vi "实时小时数据处理整合 (子VI).vi"(11 "枚举":enum16{"实时数据排序", "小时数据排序"}(ring)) -> (3 "已排序的数组":string[](array[string]))   [LabVIEW 2016, in "数据传输系统.lvlib"]
uses:
  <userlib>/_OpenG.lib/array/array.llb/Remove Duplicates from 1D Array (String)__ogtk.vi
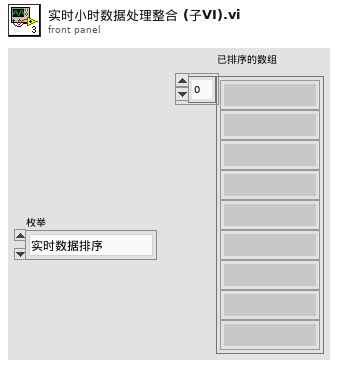
[diagram p1: front panel]
types:
  T1 = cluster{"PH":string[][], "CODCr":string[][], "氨氮":string[][], "CODMn":string[][], "总氮":string[][], "总磷":string[][], "电导率":string[][], "水温":string[][], "COD":string[][], "DO":string[][], "浊度":string[][], "叶绿素":string[][], "藻密度":string[][], "铜":string[][], "盐度":string[][], "水位":string[][], "流速":string[][], "方向":string[][], "瞬时流量":string[][], "累积流量":string[][], "正累积流量":string[][], "负累积流量":string[][], "亚硝酸盐":string[][], "硫化物":string[][], "ORP":string[][], "铅":string[][], "镉":string[][], "锌":string[][], "镍":string[][], "锰":string[][], "汞":string[][], "气温":string[][], "气压":string[][], "风速":string[][], "风向":string[][], "空气温度":string[][], "相对湿度":string[][], "分钟雨量":string[][], "小时雨量":string[][], "日雨量":string[][], "累积雨量":string[][], "盐度":string[][], "磷酸盐":string[][], "硝氮":string[][], "氟化物":string[][], "挥发酚":string[][], "氯化物":string[][], "蓝绿藻":string[][], "余氯":string[][], "综合生物毒性":string[][], "水深":string[][]}
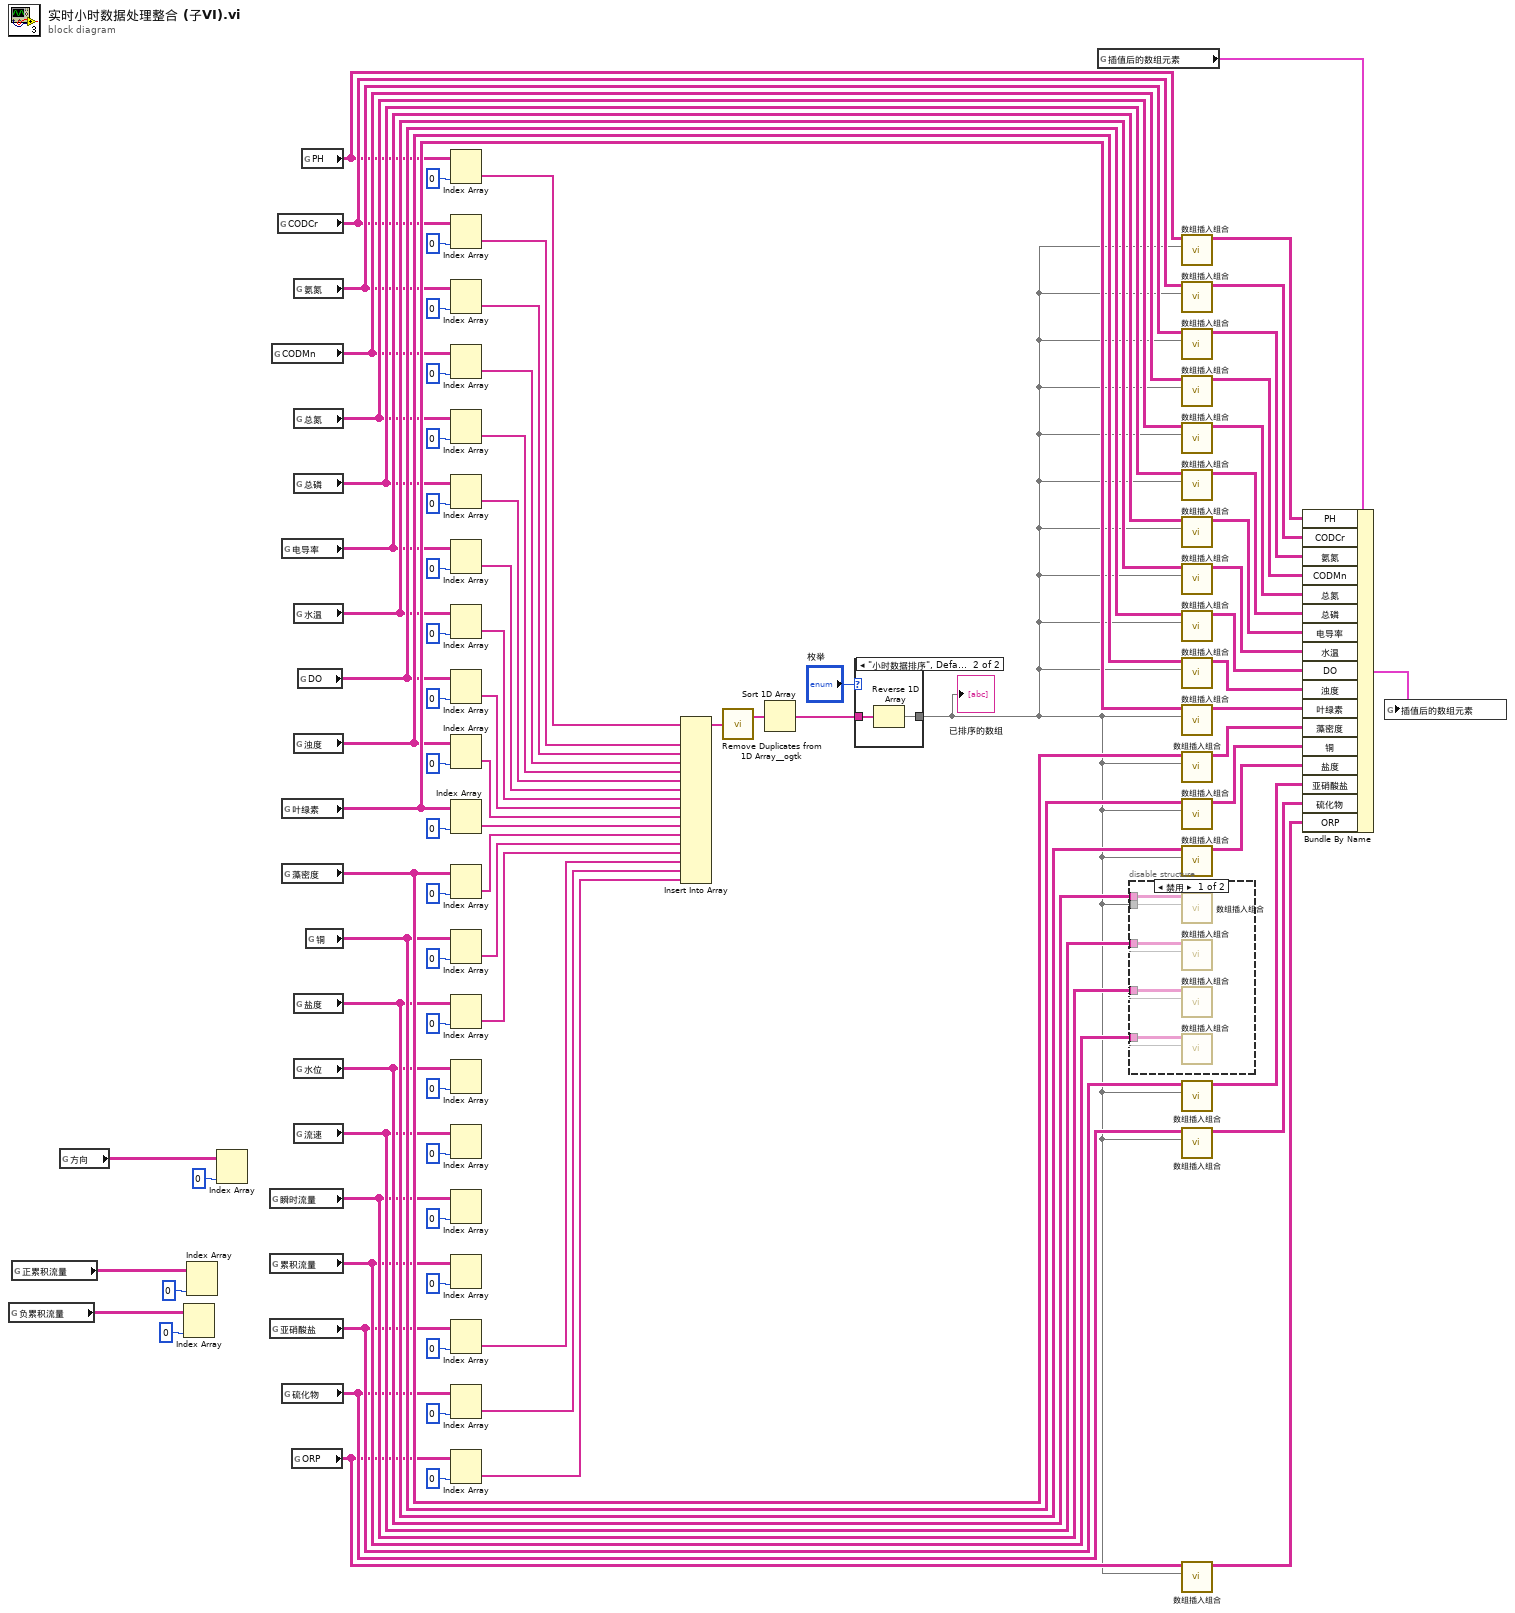
[diagram p0: block diagram]
diagram:
  n1 = global read "全局 所有参数.vi" "负累积流量"() -> (w5:string[][])
  n2 = global read "全局 所有参数.vi" "正累积流量"() -> (w6:string[][])
  n3 = global read "全局 所有参数.vi" "方向"() -> (w9:string[][])
  n4 = Index Array(array=w5, index (col)=0 ("索引 (列)")) -> ()  [unwired: 1 in, 1 out]
  n5 = Index Array(array=w6, index (col)=0 ("索引 (列)")) -> ()  [unwired: 1 in, 1 out]
  n6 = Index Array(array=w9, index (col)=0 ("索引 (列)")) -> ()  [unwired: 1 in, 1 out]
  n7 = global read "全局 所有参数.vi" "瞬时流量"() -> (w23:string[][])
  n8 = global read "全局 所有参数.vi" "累积流量"() -> (w22:string[][])
  n9 = global read "全局 所有参数.vi" "亚硝酸盐"() -> (w19:string[][])
  n10 = global read "全局 所有参数.vi" "CODMn"() -> (w70:string[][])
  n11 = global read "全局 所有参数.vi" "CODCr"() -> (w68:string[][])
  n12 = global read "全局 所有参数.vi" "电导率"() -> (w73:string[][])
  n13 = global read "全局 所有参数.vi" "叶绿素"() -> (w77:string[][])
  n14 = global read "全局 所有参数.vi" "藻密度"() -> (w78:string[][])
  n15 = global read "全局 所有参数.vi" "硫化物"() -> (w16:string[][])
  n16 = global read "全局 所有参数.vi" "ORP"() -> (w15:string[][])
  n17 = global read "全局 所有参数.vi" "氨氮"() -> (w69:string[][])
  n18 = global read "全局 所有参数.vi" "总氮"() -> (w71:string[][])
  n19 = global read "全局 所有参数.vi" "总磷"() -> (w72:string[][])
  n20 = global read "全局 所有参数.vi" "水温"() -> (w74:string[][])
  n21 = global read "全局 所有参数.vi" "浊度"() -> (w76:string[][])
  n22 = global read "全局 所有参数.vi" "盐度"() -> (w36:string[][])
  n23 = global read "全局 所有参数.vi" "水位"() -> (w28:string[][])
  n24 = global read "全局 所有参数.vi" "流速"() -> (w26:string[][])
  n25 = global read "全局 所有参数.vi" "DO"() -> (w75:string[][])
  n26 = global read "全局 所有参数.vi" "PH"() -> (w66:string[][])
  n27 = global read "全局 所有参数.vi" "铜"() -> (w37:string[][])
  n28 = Index Array(array=w66, index (col)=0 ("索引 (行)")) -> (element=w53:string[])  [unwired: 1 in]
  n29 = Index Array(array=w68, index (col)=0 ("索引 (行)")) -> (element=w54:string[])  [unwired: 1 in]
  n30 = Index Array(array=w69, index (col)=0 ("索引 (行)")) -> (element=w55:string[])  [unwired: 1 in]
  n31 = Index Array(array=w70, index (col)=0 ("索引 (行)")) -> (element=w56:string[])  [unwired: 1 in]
  n32 = Index Array(array=w71, index (col)=0 ("索引 (行)")) -> (element=w57:string[])  [unwired: 1 in]
  n33 = Index Array(array=w72, index (col)=0 ("索引 (行)")) -> (element=w58:string[])  [unwired: 1 in]
  n34 = Index Array(array=w73, index (col)=0 ("索引 (行)")) -> (element=w59:string[])  [unwired: 1 in]
  n35 = Index Array(array=w74, index (col)=0 ("索引 (行)")) -> (element=w60:string[])  [unwired: 1 in]
  n36 = Index Array(array=w75, index (col)=0 ("索引 (行)")) -> (element=w61:string[])  [unwired: 1 in]
  n37 = Index Array(array=w76, index (col)=0 ("索引 (行)")) -> (element=w62:string[])  [unwired: 1 in]
  n38 = Index Array(array=w77, index (col)=0 ("索引 (行)")) -> (element=w63:string[])  [unwired: 1 in]
  n39 = Index Array(array=w78, index (col)=0 ("索引 (行)")) -> (element=w64:string[])  [unwired: 1 in]
  n40 = Index Array(array=w37, index (col)=0 ("索引 (行)")) -> (element=w35:string[])  [unwired: 1 in]
  n41 = Index Array(array=w36, index (col)=0 ("索引 (行)")) -> (element=w34:string[])  [unwired: 1 in]
  n42 = Index Array(array=w28, index (col)=0 ("索引 (列)")) -> ()  [unwired: 1 in, 1 out]
  n43 = Index Array(array=w26, index (col)=0 ("索引 (列)")) -> ()  [unwired: 1 in, 1 out]
  n44 = Index Array(array=w23, index (col)=0 ("索引 (列)")) -> ()  [unwired: 1 in, 1 out]
  n45 = Index Array(array=w22, index (col)=0 ("索引 (列)")) -> ()  [unwired: 1 in, 1 out]
  n46 = Index Array(array=w19, index (col)=0 ("索引 (列)")) -> (element=w3:string[])  [unwired: 1 in]
  n47 = Index Array(array=w16, index (col)=0 ("索引 (列)")) -> (element=w2:string[])  [unwired: 1 in]
  n48 = Index Array(array=w15, index (col)=0 ("索引 (列)")) -> (element=w1:string[])  [unwired: 1 in]
  n49 = Insert Into Array(array=w53, new element #1=w54, new element #2=w55, new element #3=w56, new element #4=w57, new element #5=w58, new element #6=w59, new element #7=w60, new element #8=w61, new element #9=w62, new element #10=w63, new element #11=w64, new element #12=w35, new element #13=w34, new element #14=w3, new element #15=w2, new element #16=w1) -> (w65:string[])  [unwired: 1 in]
  n50 = call-poly <userlib>:"Remove Duplicates from 1D Array__ogtk.vi"("Input Array"=w65) -> ("Output Array"=w52:string[])  [unwired: 1 out]
  n51 = Sort 1D Array(array=w52) -> (sorted array=w38:string[])
  n52 = case shown="\"小时数据排序\", Default" "枚举" {
    tunnel: w38 -> [w90 w92]
    tunnel: [w90 w91] -> w12
    frame "实时数据排序" {
    }
    frame "小时数据排序", Default {
      n53 = Reverse 1D Array(array=w92) -> (reversed array=w91:string[])
    }
  }
  "已排序的数组" <- w12
  n54 = global read "插值后的新数组.vi" "插值后的数组元素"() -> (w21:T1)
  n55 = disable-structure shown="禁用" {
    disable-tunnel: w28 -> [w97 _]
    disable-tunnel: w26 -> [w96 _]
    disable-tunnel: w23 -> [w95 _]
    disable-tunnel: w22 -> [w94 _]
    disable-tunnel: w12 -> [w93 _]
    frame Disabled {
      n56 = call "数组插入组合.vi"("排序后的一维数组"=w93, "输入数组"=w97) -> ()  [unwired: 9 in, 1 out]
      n57 = call "数组插入组合.vi"("排序后的一维数组"=w93, "输入数组"=w96) -> ()  [unwired: 9 in, 1 out]
      n58 = call "数组插入组合.vi"("排序后的一维数组"=w93, "输入数组"=w95) -> ()  [unwired: 9 in, 1 out]
      n59 = call "数组插入组合.vi"("排序后的一维数组"=w93, "输入数组"=w94) -> ()  [unwired: 9 in, 1 out]
    }
    frame Enabled {
    }
  }
  n60 = call "数组插入组合.vi"("排序后的一维数组"=w12, "输入数组"=w66) -> ("输出结果"=w67:string[][])  [unwired: 9 in]
  n61 = call "数组插入组合.vi"("排序后的一维数组"=w12, "输入数组"=w68) -> ("输出结果"=w79:string[][])  [unwired: 9 in]
  n62 = call "数组插入组合.vi"("排序后的一维数组"=w12, "输入数组"=w69) -> ("输出结果"=w80:string[][])  [unwired: 9 in]
  n63 = call "数组插入组合.vi"("排序后的一维数组"=w12, "输入数组"=w70) -> ("输出结果"=w81:string[][])  [unwired: 9 in]
  n64 = call "数组插入组合.vi"("排序后的一维数组"=w12, "输入数组"=w71) -> ("输出结果"=w82:string[][])  [unwired: 9 in]
  n65 = call "数组插入组合.vi"("排序后的一维数组"=w12, "输入数组"=w72) -> ("输出结果"=w83:string[][])  [unwired: 9 in]
  n66 = call "数组插入组合.vi"("排序后的一维数组"=w12, "输入数组"=w73) -> ("输出结果"=w84:string[][])  [unwired: 9 in]
  n67 = call "数组插入组合.vi"("排序后的一维数组"=w12, "输入数组"=w74) -> ("输出结果"=w85:string[][])  [unwired: 9 in]
  n68 = call "数组插入组合.vi"("排序后的一维数组"=w12, "输入数组"=w75) -> ("输出结果"=w86:string[][])  [unwired: 9 in]
  n69 = call "数组插入组合.vi"("排序后的一维数组"=w12, "输入数组"=w76) -> ("输出结果"=w87:string[][])  [unwired: 9 in]
  n70 = call "数组插入组合.vi"("排序后的一维数组"=w12, "输入数组"=w77) -> ("输出结果"=w88:string[][])  [unwired: 9 in]
  n71 = call "数组插入组合.vi"("排序后的一维数组"=w12, "输入数组"=w78) -> ("输出结果"=w89:string[][])  [unwired: 9 in]
  n72 = call "数组插入组合.vi"("排序后的一维数组"=w12, "输入数组"=w37) -> ("输出结果"=w33:string[][])  [unwired: 9 in]
  n73 = call "数组插入组合.vi"("排序后的一维数组"=w12, "输入数组"=w36) -> ("输出结果"=w32:string[][])  [unwired: 9 in]
  n74 = call "数组插入组合.vi"("排序后的一维数组"=w12, "输入数组"=w19) -> ("输出结果"=w10:string[][])  [unwired: 9 in]
  n75 = call "数组插入组合.vi"("排序后的一维数组"=w12, "输入数组"=w16) -> ("输出结果"=w11:string[][])  [unwired: 9 in]
  n76 = call "数组插入组合.vi"("排序后的一维数组"=w12, "输入数组"=w15) -> ("输出结果"=w13:string[][])  [unwired: 9 in]
  n77 = Bundle By Name(cluster=w21, "PH"=w67, "CODCr"=w79, "氨氮"=w80, "CODMn"=w81, "总氮"=w82, "总磷"=w83, "电导率"=w84, "水温"=w85, "DO"=w86, "浊度"=w87, "叶绿素"=w88, "藻密度"=w89, "铜"=w33, "盐度"=w32, "亚硝酸盐"=w10, "硫化物"=w11, "ORP"=w13) -> (w20:T1)
  n78 = global write "插值后的新数组.vi" "插值后的数组元素"(w20) -> ()
